vi "F Dwf Analog Out Data Set.vi"(7 "cdData":i32, 8 "error in (no error)":errorcluster, 9 "rgdData":dbl[](array[numeric]), 10 "idxChannel":i32, 11 "hdwf":i32) -> (0 "error out":errorcluster, 3 "function return":i32)   [LabVIEW 2019, in "Olasdwf.lvlib"]
doc: "DWFAPI int FDwfAnalogOutDataSet(HDWF hdwf, int idxChannel, double *rgdData, int cdData);"
uses:
  Olasdwf.lvlib
  Windows/System32/dwf.dll
panel:
  out "rgdData 2":dbl[](array[numeric])
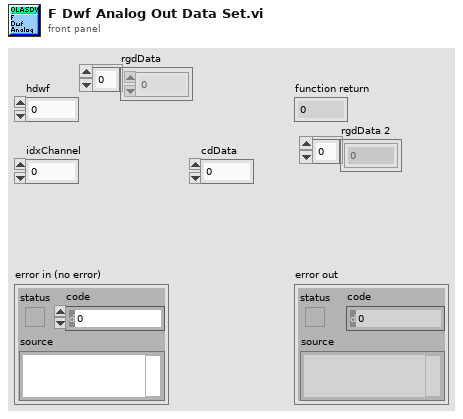
[diagram p1: front panel]
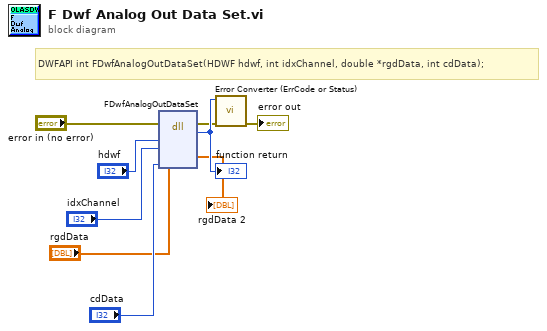
[diagram p0: block diagram]
diagram:
  # "DWFAPI int FDwfAnalogOutDataSet(HDWF hdwf, int idxChannel, double *rgdData, int cdData);"
  n1 = dll-call lib="C:/Windows/System32/dwf.*" fn="FDwfAnalogOutDataSet"(error in="error in (no error)", "hdwf"="hdwf", "idxChannel"="idxChannel", "rgdData"="rgdData", "cdData"="cdData") -> (error out=w4:errorcluster, "return type"=w9:i32, "rgdData"=→"rgdData 2":dbl[])  [unwired: 5 in, 1 out]
  "function return" <- w9
  n2 = call "Error Converter (ErrCode or Status).vi"("error in (no error)"=w4, "error code"=w9) -> ("error out"=→"error out":errorcluster)  [unwired: 9 in]
